vi "main.vi"(9 "handler properties":T1={"max url size"=8000, "max header"=8000, "timeout ms"=15000, "max data size"=104857600}, 10 "connection handler pool size":i32=10, 11 "port":u16=443) -> (0 "error out":errorcluster)   [LabVIEW 2016]
uses:
  HTTP server/http server properties.ctl
  tests/ws console/Websocket console plugin.lvclass
  C:/Users/IEUser/Desktop/http/websocket/user plugin/websocket user plugin.lvclass
  tests/test responder/test responder.lvclass
  C:/Users/IEUser/Desktop/http/HTTP responder/http responder.lvclass
  TLS HTTP server/TLS HTTP server.lvclass/TLS HTTP server.ctl
  TLS HTTP server/Read lvlibretls server listener.vi
  TLS HTTP server/Write lvlibretls server listener.vi
  TLS HTTP server/TLS HTTP server.lvclass
  C:/Users/IEUser/Desktop/http/HTTP server/Basic HTTP server.lvclass
  lvlibtls/server/lvlibretls server listener.lvclass
  C:/Users/IEUser/Desktop/http/lvlibtls/context parent/lvlibretls configurable context.lvclass
  HTTP responder/http responder.lvclass
  websocket/websocket upgrade handler.lvclass
  HTTP server/Basic HTTP server.lvclass
  lvlibtls/context parent/lvlibretls configurable context.lvclass
panel:
  in  "stop":bool
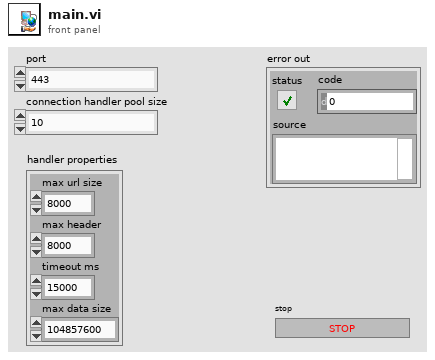
[diagram p1: front panel]
types:
  T1 = typedef "Basic HTTP server.lvclass/http server properties.ctl" = cluster{"max url size":i32, "max header":i32, "timeout ms":i32, "max data size":i32}
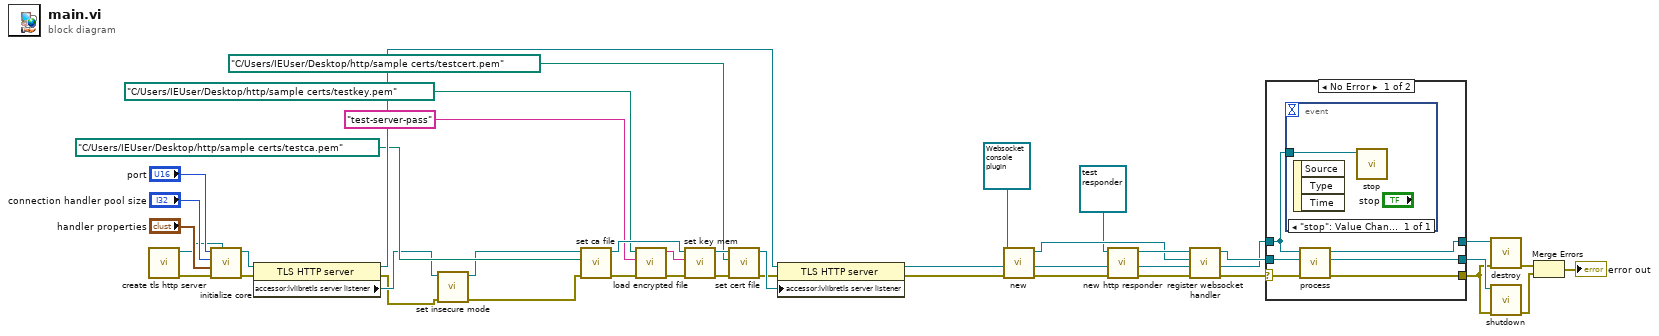
[diagram p0: block diagram]
diagram:
  n1 = call "create tls http server.vi"() -> ("error out"=w22:errorcluster, "TLS HTTP server out"=w21:refnum<class "TLS HTTP server.lvclass">)  [unwired: 10 in]
  n2 = call "initialize core.vi"("specialization"=w21, "error in"=w22, "handler properties"="handler properties", "connection handler pool size"="connection handler pool size", "port"="port") -> ("error out"=w32:errorcluster, "Basic HTTP server out"=w20:refnum<class "TLS HTTP server.lvclass">)  [unwired: 5 in]
  n3 = property class="TLS HTTP server"(reference=w20, error in=w32) -> (reference out=w18:refnum<class "TLS HTTP server.lvclass">, error out=w3:errorcluster, "accessor:lvlibretls server listener"=w4:refnum<class "lvlibretls server listener.lvclass">)
  n4 = call "set insecure mode.vi"("error in"=w3, "lvlibretls configurable context in"=w4) -> ("error out"=w2:errorcluster, "lvlibretls configurable context out"=w1:refnum<class "lvlibretls server listener.lvclass">)  [unwired: 8 in]
  n5 = call "set ca file.vi"("error in"=w2, "ca file"=path "C:/Users/IEUser/Desktop/http/sample certs/testca.pem", "lvlibretls configurable context in"=w1) -> ("error out"=w11:errorcluster, "lvlibretls configurable context out"=w10:refnum<class "lvlibretls server listener.lvclass">)  [unwired: 7 in]
  n6 = call "load encrypted file.vi"("error in"=w11, "password"="test-server-pass", "Path"=path "C:/Users/IEUser/Desktop/http/sample certs/testkey.pem" ("key file")) -> ("error out"=w14:errorcluster, "data"=w15:string)  [unwired: 7 in]
  n7 = call "set key mem.vi"("error in"=w14, "key file"=w15, "lvlibretls configurable context in"=w10) -> ("error out"=w12:errorcluster, "lvlibretls configurable context out"=w13:refnum<class "lvlibretls server listener.lvclass">)  [unwired: 7 in]
  n8 = call "set cert file.vi"("error in"=w12, "cert file"=path "C:/Users/IEUser/Desktop/http/sample certs/testcert.pem" ("ca file"), "lvlibretls configurable context in"=w13) -> ("error out"=w5:errorcluster, "lvlibretls configurable context out"=w6:refnum<class "lvlibretls server listener.lvclass">)  [unwired: 7 in]
  n9 = property class="TLS HTTP server"(reference=w18, error in=w5, "accessor:lvlibretls server listener"=w6) -> (reference out=w17:refnum<class "TLS HTTP server.lvclass">, error out=w19:errorcluster)
  n10 = call-dynamic "new.vi"("error in"=w19, "Websocket console plugin in"=refnum<class "Websocket console plugin.lvclass"> refnum ("Websocket console plugin")) -> ("error out"=w28:errorcluster, "Websocket console plugin out"=w25:refnum<class "Websocket console plugin.lvclass">)  [unwired: 8 in]
  n11 = call-dynamic "new http responder.vi"("error in"=w28, "http responder in"=refnum<class "test responder.lvclass"> refnum ("test responder.lvclass")) -> ("error out"=w30:errorcluster, "http responder out"=w26:refnum<class "test responder.lvclass">)  [unwired: 8 in]
  n12 = call "register websocket handler.vi"("error in"=w30, "websocket user plugin"=w25, "http responder in"=w26) -> ("error out"=w29:errorcluster, "http responder out"=w27:refnum<class "test responder.lvclass">)  [unwired: 7 in]
  n13 = case shown="No Error" w29 {
    selector: w29 -> [w43 w49]
    tunnel: w17 -> [w46 w50]
    tunnel: [w45 w50] -> w37
    tunnel: [w44 w48] -> w36
    tunnel: w27 -> [w42 w48]
    tunnel: [w41 w49] -> w31
    frame No Error {
      n14 = event shown="[0] \"stop\": Value Change" {
        selector: _ -> [_]
        dyn-events: _ -> [_]
        timeout: _ -> [_]
        tunnel: w46 -> [w47]
        event "stop": Value Change {
          n15 = event-data() -> ()  [unwired: 1 in, 3 out]
          n16 = call "stop.vi"("Basic HTTP server in"=w47) -> ()  [unwired: 10 in, 1 out]
        }
      }
      n17 = call "process.vi"("error in"=w43, "responder in"=w42, "Basic HTTP server in"=w46) -> ("error out"=w41:errorcluster, "responder out"=w44:refnum<class "test responder.lvclass">, "Basic HTTP server out"=w45:refnum<class "TLS HTTP server.lvclass">)  [unwired: 6 in]
    }
    frame Error {
    }
  }
  n18 = call-dynamic "destroy.vi"("error in"=w31, "TLS HTTP server in"=w37) -> ("error out"=w33:errorcluster)  [unwired: 9 in]
  n19 = call "shutdown.vi"("error in"=w31, "http responder in"=w36) -> ("error out"=w34:errorcluster)  [unwired: 9 in]
  n20 = Merge Errors(w33, w34) -> (→"error out":errorcluster)
